vi "loading.vi"(3 "error in":errorcluster, 4 "Message":string, 5 "Pop-up Type":T1(ring)) -> (0 "error out":errorcluster)   [LabVIEW 2019, in "ZenGage v3.0 UI.lvclass"]
uses:
  ZenGage v3.0 UI.lvclass
panel:
  out "loading message":string="LOGIN STATUS......"
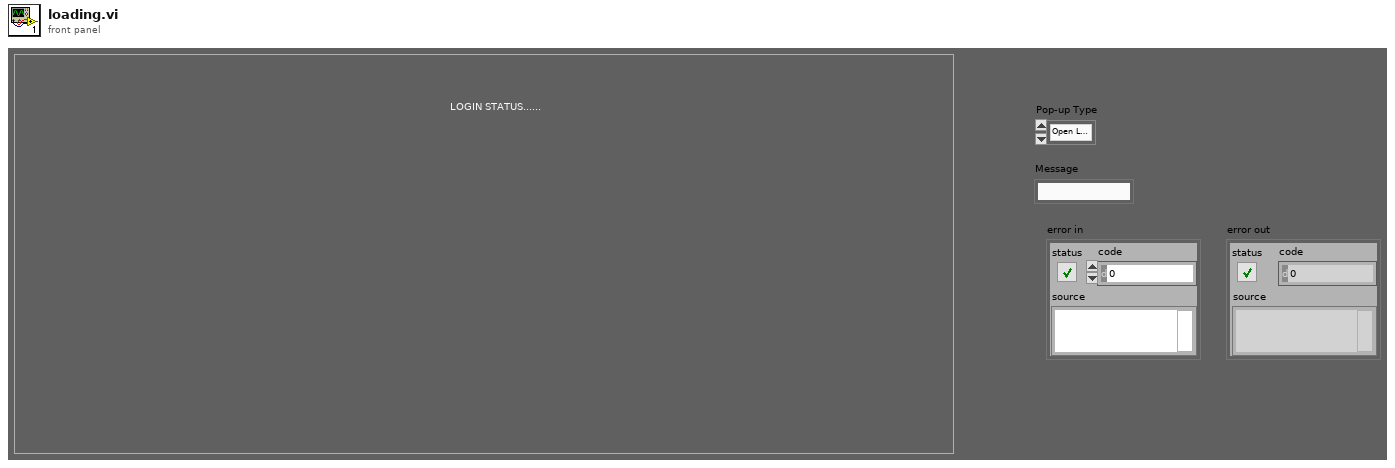
[diagram p1: front panel]
types:
  T1 = enum16{"Open Logo Display", "Close Logo Display", "Open Loading Bar", "Close Loading Bar", "Open Alert Display", "Close Alert Display", "One button dialog box", "Two button dialog box", "User Authentication"}
  T2 = enum32{"Invalid", "Standard", "Closed", "Hidden", "Minimized", "Maximized"}
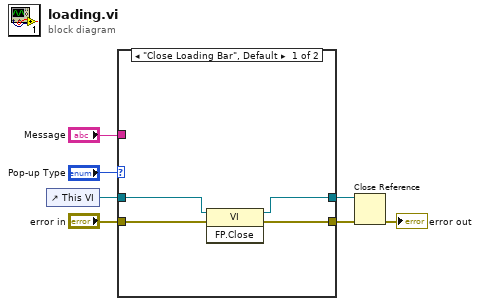
[diagram p0: block diagram]
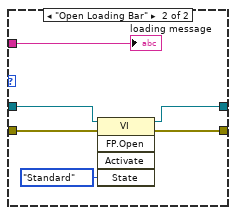
[diagram p2: hidden frame]
diagram:
  n1 = control-ref of="This VI"() -> (w6:refnum<vi>)
  n2 = case shown="\"Close Loading Bar\", Default" "Pop-up Type" {
    tunnel: [w10 w16] -> w5
    tunnel: "error in" -> [w11 w17]
    tunnel: w6 -> [w9 w15]
    tunnel: [w8 w14] -> w3
    tunnel: "Message" -> [_ w13]
    frame "Close Loading Bar", Default {
      n3 = invoke class="VI" method="FP.Close"(reference=w9, error in=w11) -> (reference out=w8:refnum<vi>, error out=w10:errorcluster)  [unwired: 1 in, 1 out]
    }
    frame "Open Loading Bar" {
      n4 = invoke class="VI" method="FP.Open"(reference=w15, error in=w17, "State"=T2."Standard") -> (reference out=w14:refnum<vi>, error out=w16:errorcluster)  [unwired: 2 in, 3 out]
      "loading message" <- w13
    }
  }
  n5 = Close Reference(reference=w3, error in (no error)=w5) -> (error out=→"error out":errorcluster)
